vi "RenameMembers.vi"(8 "error in (no error)":errorcluster, 9 "ReplaceString":string, 10 "SearchString":string, 11 "LVClassLibrary Refnum":refnum<vi>) -> (0 "error out":errorcluster, 3 "Library Refnum out":refnum<vi>)   [LabVIEW 2014, in "ClassRenamer.lvclass"]
uses:
  ClassRenamer.lvclass
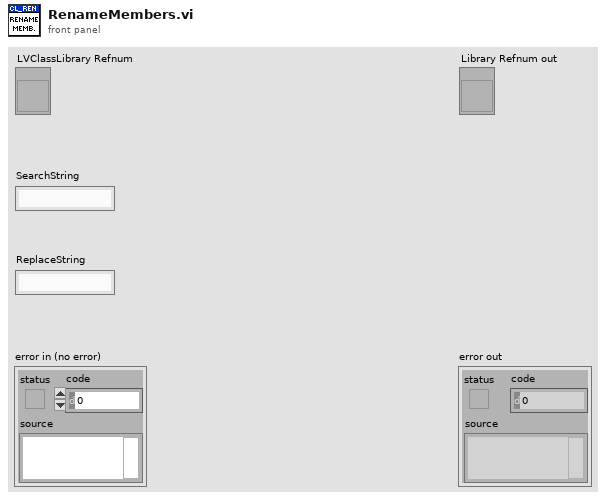
[diagram p1: front panel]
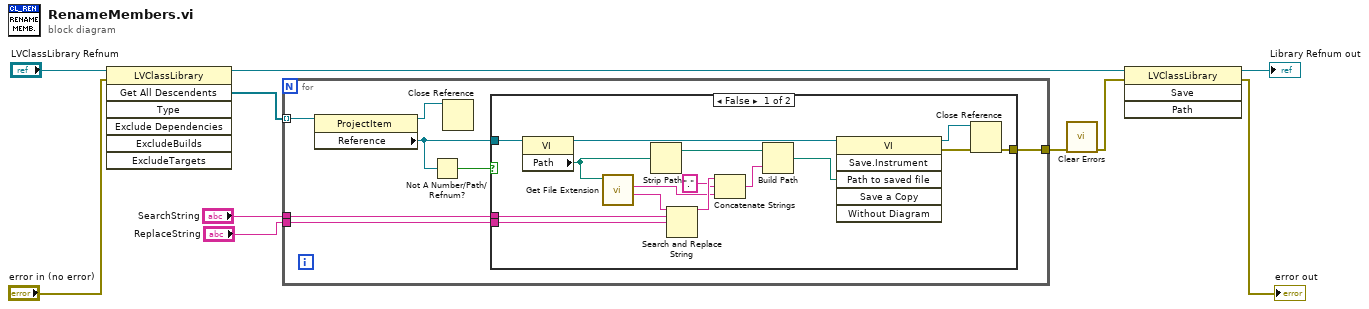
[diagram p0: block diagram]
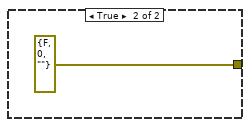
[diagram p2: hidden frame]
diagram:
  n1 = invoke class="LVClassLibrary" method="Get All Descendents"(reference="LVClassLibrary Refnum", error in="error in (no error)") -> (reference out=w3:refnum<vi>, "All Descendents"=w5:refnum<vi>[])  [unwired: 5 in, 5 out]
  n2 = for {
    tunnel: w5 -> [w17] mode=indexing
    tunnel: "SearchString" -> [w13]
    tunnel: "ReplaceString" -> [w12]
    tunnel: [w11] -> w8
    n3 = property class="ProjectItem"(reference=w17) -> (reference out=w14:refnum<vi>, "Reference"=w15:refnum<vi>)  [unwired: 1 in, 1 out]
    n4 = Not A Number/Path/Refnum?(number/path/refnum=w15) -> (NaN/Path/Refnum?=w16:bool)
    n5 = Close Reference(reference=w14) -> ()  [unwired: 1 in, 1 out]
    n6 = case shown="False" w16 {
      tunnel: w15 -> [w32 _]
      tunnel: w13 -> [w30 _]
      tunnel: w12 -> [w29 _]
      tunnel: [w19 errorcluster {"status"=FALSE, "code"=0, "source"=""} ("error out")] -> w11
      frame False {
        n7 = property class="VI"(reference=w32) -> (reference out=w28:refnum<vi>, "Path"=w27:path)  [unwired: 1 in, 1 out]
        n8 = call <vilib>:"Get File Extension.vi"("file"=w27) -> ("filename without extension"=w31:string, "lowercase file extension"=w25:string)  [unwired: 7 in, 2 out]
        n9 = Strip Path(path=w27) -> (stripped path=w24:path)  [unwired: 1 out]
        n10 = Search and Replace String(input string=w31, search string=w30, replace string=w29) -> (result string=w26:string)  [unwired: 5 in, 3 out]
        n11 = Concatenate Strings(w26, "." ("string"), w25) -> (w23:string)
        n12 = Build Path(base path=w24, name or relative path=w23) -> (appended path=w22:path)
        n13 = invoke class="VI" method="Save.Instrument"(reference=w28, "Path to saved file"=w22) -> (reference out=w20:refnum<vi>, error out=w21:errorcluster)  [unwired: 4 in, 4 out]
        n14 = Close Reference(reference=w20, error in (no error)=w21) -> (error out=w19:errorcluster)
      }
      frame True {
      }
    }
  }
  n15 = call <vilib>:"Clear Errors.vi"("error in (no error)"=w8) -> ("error out"=w10:errorcluster)  [unwired: 5 in, 1 out]
  n16 = invoke class="LVClassLibrary" method="Save"(reference=w3, error in=w10) -> (reference out=→"Library Refnum out":refnum<vi>, error out=→"error out":errorcluster)  [unwired: 2 in, 2 out]
